vi "ReadMultiPoint.vi"(8 "error in (no error)":errorcluster, 11 "NiPxi6123 in":refnum<class "NiPxi6123.lvclass">) -> (0 "error out":errorcluster, 3 "NiPxi6123 out":refnum<class "NiPxi6123.lvclass">)   [LabVIEW 2014, in "SamplerPlugins.lvlib" / "NiPxi6123.lvclass"]
uses:
  NiPxi6123.lvclass
  <vilib>/DAQmx/read.llb/DAQmx Read (Analog 2D DBL NChan NSamp).vi
  <vilib>/DAQmx/configure/trigger.llb/DAQmx Start Trigger (Digital Edge).vi
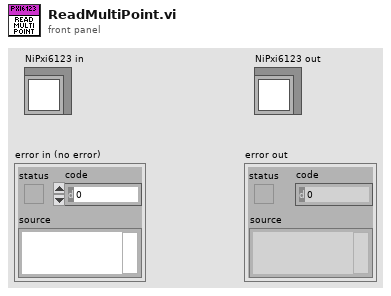
[diagram p1: front panel]
types:
  T1 = typedef "SamplerPlugins.lvlib/SamplerPluginsBase.lvclass/ReadMultiPointParams.ctl" = cluster{"iMaxTimeMilliseconds":i32, "iArraySize":i32}
  T2 = typedef "SamplerPlugins.lvlib/SamplerPluginsBase.lvclass/ConfigMultiPointParams.ctl" = cluster{"iTriggerCount":i32, "iSampleCount":i32, "eSampleClock":u16, "dSampleInterval":dbl}
  T3 = typedef "NISTSamplerPlugins.lvlib/NISTSamplerPluginsBase.lvclass/TriggerParams.ctl" = cluster{"eEdge":u16, "sSource":string}
  T4 = typedef "SamplerPlugins.lvlib/SamplerPluginsBase.lvclass/MultiPointReadingArrayParams.ctl" = T5[]
  T5 = typedef "SamplerPlugins.lvlib/SamplerPluginsBase.lvclass/MultiPointReadingParams.ctl" = cluster{"dReadingArray":dbl[], "iActualPts":i32, "Timestamp":dbl}
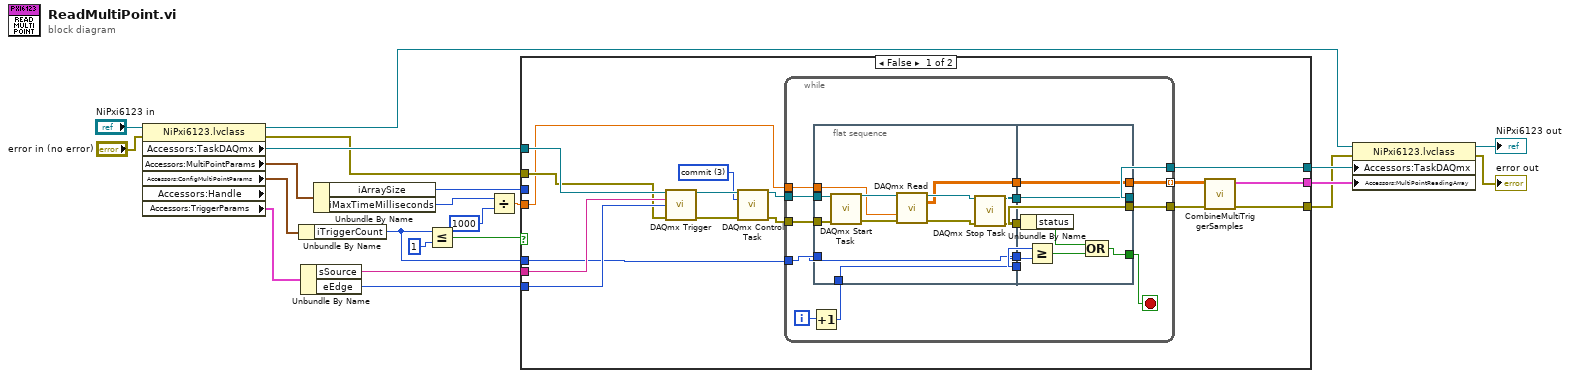
[diagram p0: block diagram]
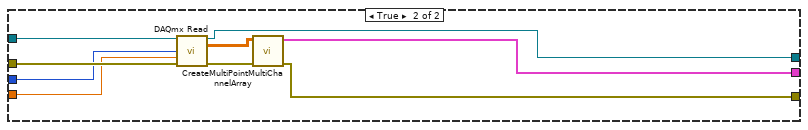
[diagram p2: hidden frame]
diagram:
  n1 = property class="NiPxi6123.lvclass" props=["Accessors:TaskDAQmx", "Accessors:MultiPointParams", "Accessors:ConfigMultiPointParams", "Accessors:Handle", "Accessors:TriggerParams"](reference="NiPxi6123 in", error in="error in (no error)") -> (reference out=w11:refnum<class "NiPxi6123.lvclass">, error out=w19:errorcluster, "Accessors:TaskDAQmx"=w20:refnum<k21>, "Accessors:MultiPointParams"=w18:T1, "Accessors:ConfigMultiPointParams"=w10:T2, "Accessors:TriggerParams"=w7:T3)  [unwired: 1 out]
  n2 = Unbundle By Name(w10) -> ("iTriggerCount"=w4:i32)
  n3 = Unbundle By Name(w7) -> ("sSource"=w6:string, "eEdge"=w5:u16)
  n4 = Unbundle By Name(w18) -> ("iArraySize"=w17:i32, "iMaxTimeMilliseconds"=w2:i32)
  n5 = Less Or Equal?(x=w4, y=1) -> (x <= y?=w8:bool)
  n6 = Divide(x=w2, y=1000) -> (x/y=w1:dbl)
  n7 = case shown="False" w8 {
    tunnel: w20 -> [w36 w82]
    tunnel: w19 -> [w35 w81]
    tunnel: w17 -> [_ w80]
    tunnel: w1 -> [w23 w79]
    tunnel: [w31 w76] -> w16
    tunnel: [w33 w78] -> w15
    tunnel: [w34 w74] -> w14
    tunnel: w6 -> [w38 _]
    tunnel: w5 -> [w37 _]
    tunnel: w4 -> [w32 _]
    frame False {
      w28 = 3 items=["verify"=2, "reserve"=4, "commit"=3, "unreserve"=5, "abort"=6] ("action")
      n8 = call-poly <vilib>:"DAQmx Trigger.vi"("task/channels in"=w36, "source"=w38, "edge"=w37, "error in"=w35) -> ("task out"=w30:refnum<k21>, "error out"=w29:errorcluster)  [unwired: 10 in]
      n9 = call <vilib>:"DAQmx Control Task.vi"("task/channels in"=w30, "action"=w28, "error in"=w29) -> ("task out"=w27:refnum<k21>, "error out"=w26:errorcluster)  [unwired: 11 in]
      n10 = while {
        tunnel: w27 -> [w53]
        tunnel: w26 -> [w52]
        tunnel: [w48] -> w33
        tunnel: w32 -> [w46]
        tunnel: [w43] -> w25 mode=indexing
        tunnel: [w42] -> w24
        tunnel: w23 -> [w39]
        i -> [w41]
        stop <- w50 stop-if-true
        n11 = Increment(x=w41) -> (x+1=w40:i32)
        n12 = flat-sequence {
          tunnel: w53 -> [w65]
          tunnel: w52 -> [w64]
          tunnel: [w59] -> w51
          tunnel: [w58] -> w49
          tunnel: w40 -> [w57]
          tunnel: [w57] -> w47
          tunnel: w46 -> [w56]
          tunnel: [w56] -> w45
          tunnel: [w55] -> w44
          tunnel: w39 -> [w54]
          tunnel: w51 -> [w66]
          tunnel: [w68] -> w50
          tunnel: w49 -> [w73]
          tunnel: [w73] -> w48
          tunnel: w47 -> [w72]
          tunnel: w45 -> [w71]
          tunnel: w44 -> [w67]
          tunnel: [w67] -> w43
          tunnel: [w66] -> w42
          frame #0 {
            n13 = call <vilib>:"DAQmx Start Task.vi"("task/channels in"=w65, "error in"=w64) -> ("task out"=w63:refnum<k21>, "error out"=w62:errorcluster)  [unwired: 12 in]
            n14 = call-poly <vilib>:"DAQmx Read.vi"("task/channels in"=w63, "timeout"=w54, "error in"=w62) -> ("task out"=w61:refnum<k21>, "data"=w55:dbl[][], "error out"=w60:errorcluster)  [unwired: 10 in]
            n15 = call <vilib>:"DAQmx Stop Task.vi"("task/channels in"=w61, "error in"=w60) -> ("task out"=w58:refnum<k21>, "error out"=w59:errorcluster)  [unwired: 12 in]
          }
          frame #1 {
            n16 = Unbundle By Name(w66) -> ("status"=w70:bool)
            n17 = Greater Or Equal?(x=w72, y=w71) -> (x >= y?=w69:bool)
            n18 = Compound Arithmetic op=OR(w70, w69) -> (w68:bool)
          }
        }
      }
      n19 = call "CombineMultiTriggerSamples.vi"("error in (no error)"=w24, "SampleArraysIn"=w25) -> ("error out"=w34:errorcluster, "MultiPointReadingArrayOut"=w31:T4)  [unwired: 8 in]
    }
    frame True {
      n20 = call-poly <vilib>:"DAQmx Read.vi"("task/channels in"=w82, "number of samples per channel"=w80, "timeout"=w79, "error in"=w81) -> ("task out"=w78:refnum<k21>, "data"=w77:dbl[][], "error out"=w75:errorcluster)  [unwired: 9 in]
      n21 = call "CreateMultiPointMultiChannelArray.vi"("error in (no error)"=w75, "MultiChannelSamplesIn"=w77) -> ("error out"=w74:errorcluster, "MultiPointReadingArrayOut"=w76:T4)  [unwired: 8 in]
    }
  }
  n22 = property class="NiPxi6123.lvclass"(reference=w11, error in=w14, "Accessors:TaskDAQmx"=w15, "Accessors:MultiPointReadingArray"=w16) -> (reference out=→"NiPxi6123 out":refnum<class "NiPxi6123.lvclass">, error out=→"error out":errorcluster)
